vi "FPGA IO.vi"() -> ()   [LabVIEW 2013]
uses:
  Reusable/PAS/Main/Controls/Laser Modulation.ctl
  <vilib>/rvi/eio/common/nirviEmuClasses.ctl
  <vilib>/Platform/TimedLoop/XDataNode/timing_clust.ctl
  <vilib>/Platform/TimedLoop/XDataNode/nitl_modes.ctl
  <vilib>/Platform/TimedLoop/XDataNode/wakeup.ctl
  <vilib>/rvi/FXPMathLib/basic elements/FxpIntAccumulator/subVIs/nifxpmath_IntAccumulator_SimConfig.ctl
  <vilib>/rvi/Emulation/niFpgaSctlEmulationGetInTimedLoop.vi
  <vilib>/rvi/Emulation/niFpgaEmulationReportErrorSimple.vi
  <vilib>/rvi/Emulation/niFpgaGetClockAttributes.vi
  <vilib>/rvi/eio/common/nirviEmuTemplateMethod_errors.vi
  <vilib>/rvi/Emulation/niFpgaProcessEmulError.vi
  <vilib>/rvi/DataTransferAndStorage/Register/Emulation/niFpgaRegisterEmulationFpgaImpl.vi
  <instcachedir>/0/niFpgaRegisterEmulationFpgaImpl_DCF4BC0110594B98B44A971D60CEEC4D.lvgen/niFpgaRegisterEmulationFpgaImpl_DCF4BC0110594B98B44A971D60CEEC4D_001.vi
  <vilib>/rvi/DataTransferAndStorage/Container/Common/niFpgaContainerGetUniqueNameForEmu.vi
  <vilib>/rvi/Emulation/niFpgaCriticalErrorInLSC.vi
  <vilib>/rvi/FXPMathLib/basic elements/FxpIntAccumulator/simVIs/DllFxpIntAccumulator_sub.vi
  <vilib>/eio/EIOGrowableMethodNode/genericMethod/EIOGrowableMethodNode.xnode
  <vilib>/rvi/eio/nirviEIOMethodImplementation/nirviEIOMethodImplementation.xnode
  <vilib>/rvi/eio/nirviErrorMerge/nirviErrorMerge.xnode
  <vilib>/rvi/DataTransferAndStorage/Container/XNode/niFpgaContainer.xnode
  <vilib>/rvi/DataTransferAndStorage/Register/Emulation/niFpgaRegisterEmulation.vi
  <vilib>/rvi/FXPMathLib/FxpMul/XNode/nifxpmath_Multiplier.xnode
  <vilib>/rvi/FXPMathLib/FxpAdd/XNode/nifxpmath_Add.xnode
  <vilib>/eio/EIONode/EIONode.xnode
  <vilib>/Platform/TimedLoop/XDataNode/XDataNode.xnode
  <vilib>/rvi/FXPMathLib/basic elements/FxpIntAccumulator/XNode/nifxpmath_IntAccumulator.xnode
  <vilib>/rvi/FXPMathLib/basic elements/FxpDiscreteDelay/XNode/nifxpmath_DiscreteDelay.xnode
  <vilib>/rvi/FXPMathLib/sim/FxpSim.dll
  <vilib>/Platform/TimedLoop/XDataNode/XDNodeRunTimeDep.lvlib
panel:
  out "PAS AO":i16
  in  "Wave":T2={"f0"=3.2499898225069046e-05, "Mod"=enum."Sine", "hrange"=0.9999999997671694, "Offset"=0} {"f0" format="%.3g"}
  in  "Speaker":cluster{"Voltage":fxp<+,14,1>, "Offset":i16}={"Voltage"=1.0, "Offset"=0}
  out "HK Data":fxp<+/-,16,5>[](array[numeric])
  out "Valves In":u8
  in  "Enables":u8
  in  "Valves Out":u8
  in  "Stop":bool
  out "Timed Out":bool
  out "Stopped":bool
  out "Error Out":errorcluster
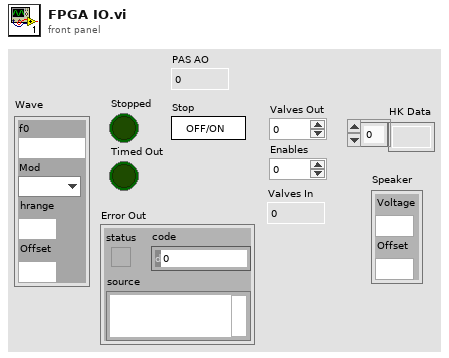
[diagram p1: front panel]
types:
  T1 = typedef "Laser Modulation.ctl" = enum8{"Sine", "Square"}
  T2 = cluster{"f0":fxp<+,32,0>, "Mod":T1, "hrange":fxp<+,32,0>, "Offset":i16}
  T3 = typedef "nirviEmuClasses.ctl" = enum16{"IO Read", "IO Write", "Method", "Property Read", "Property Write"}
  T4 = typedef "XDNodeRunTimeDep.lvlib/timing_clust.ctl" = cluster{"Expected End [f-1]":u64, "Actual End [f-1]":u64, "Finished Late? [f-1]":bool, "Expected End [i-1]":u64, "Actual End [i-1]":u64, "Finished Late? [i-1]":bool, "Expected Start [i]":u64, "Actual Start [i]":u64, "Expected Start [f]":u64, "Actual Start [f]":u64, "Source Name":string, "Structure Name":string, "Period":i64, "Deadline":i64, "Offset":i64, "Start":i64, "Priority":i32, "Timeout":i32, "Mode":T5, "Wakeup Reason":T6, "Error":errorcluster, "Source Type":string, "Secondary Source Type":string, "Global End Time":u64, "Global Start Time":u64, "Frame Duration":u64, "Iteration Duration":u64, "Assigned CPU":i32, "I/O Scan Engine Mode":u32}
  T5 = typedef "XDNodeRunTimeDep.lvlib/nitl_modes.ctl" = enum32{"No Change", "Process missed periods, maintain original phase", "Discard missed periods, maintain original phase", "Process missed periods, ignore original phase", "Discard missed periods, ignore original phase"}
  T6 = typedef "XDNodeRunTimeDep.lvlib/wakeup.ctl" = enum32{"Normal", "Aborted", "Asynchronous wakeup", "Timing source error", "Timed loop error", "Timeout"}
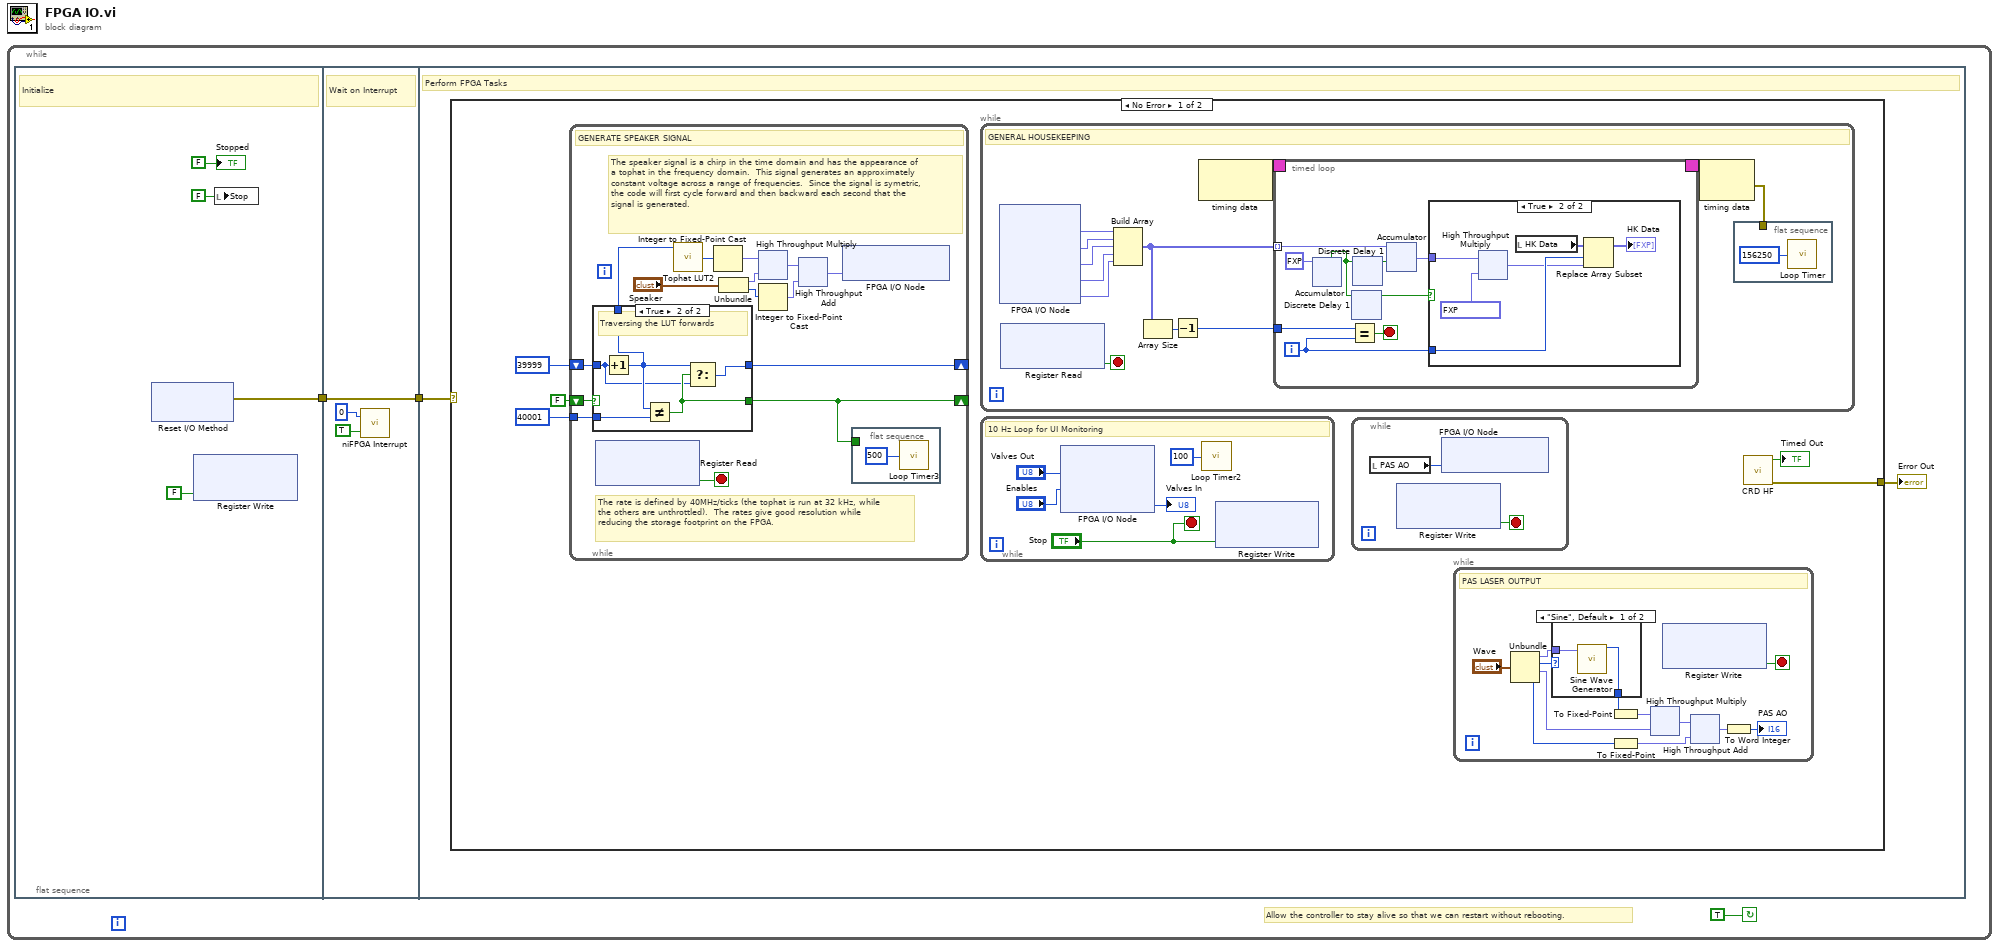
[diagram p0: block diagram]
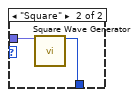
[diagram p2: hidden frame]
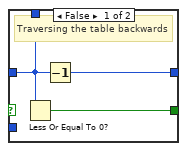
[diagram p3: hidden frame]
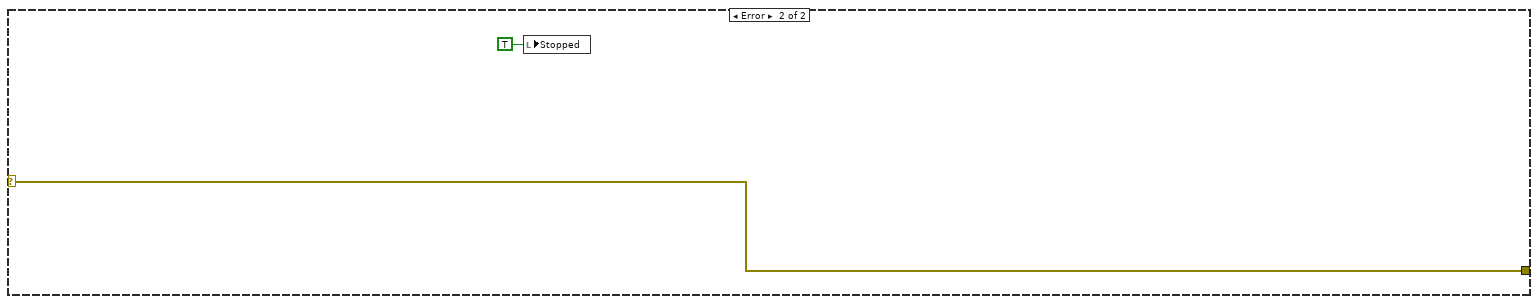
[diagram p5: hidden frame]
diagram:
  n1 = while {
    stop <- TRUE continue-if-true
    # "Allow the controller to stay alive so that we can restart without rebooting."
    n2 = flat-sequence {
      tunnel: [w6] -> w3
      tunnel: w3 -> [w52]
      tunnel: [w52] -> w2
      tunnel: w2 -> [w56]
      frame #0 {
        # "Initialize"
        n3 = xnode "Reset I/O Method"() -> ("error out"=w6:errorcluster)  [unwired: 2 in, 1 out]
        n4 = xnode ("Register Write")("Data"=FALSE) -> ()  [unwired: 1 in, 1 out]
        n5 = local write "Stop"(FALSE ("Stop")) -> ()
        "Stopped" <- FALSE ("Stopped")
      }
      frame #1 {
        # "Wait on Interrupt"
        n6 = call <vilib>:"niFPGA Interrupt.vi"("Wait Until Cleared (F)"=TRUE ("Wait Until Cleared"), "IRQ Number (0)"=u8 0 ("IRQ Number")) -> ()  [unwired: 1 in]
      }
      frame #2 {
        # "Perform FPGA Tasks"
        n7 = case shown="No Error" w56 {
          selector: w56 -> [_ w196]
          tunnel: [w61 w196] -> w55
          frame No Error {
            n8 = while {
              shift-right: [w82] -> _
              shift-left: FALSE -> [w94]
              shift-right: [w83] -> _
              shift-left: u16 39999 -> [w84]
              tunnel: u16 40001 ("y") -> [w85]
              stop <- w81 stop-if-true
              # "The rate is defined by 40MHz/ticks (the tophat is run at 32 kHz, while the others are unthrottled).  The rates give good resolution while reducing the storage footprint on the FPGA."
              # "The speaker signal is a chirp in the time domain and has the appearance of a tophat in the frequency domain.  This signal generates an approximately constant voltage across a range of frequencies.  Since the signal is symetric, the code will first cycle forward and then backward each second that the signal is generated."
              # "GENERATE SPEAKER SIGNAL"
              n9 = case "Check where we are in the chirp" shown="True" w94 {
                tunnel: w84 -> [w98 w99]
                tunnel: [w97 w102] -> w82
                tunnel: [w96 w103] -> w89
                tunnel: w85 -> [_ w101]
                tunnel: [w96 w100] -> w83
                frame False {
                  # "Traversing the table backwards"
                  n10 = Decrement(x=w98) -> (x-1=w96:u16)
                  n11 = Less Or Equal To 0?(x=w96) -> (x <= 0?=w97:bool)
                }
                frame True {
                  # "Traversing the LUT forwards"
                  n12 = Increment(x=w99) -> (x+1=w103:u16)
                  n13 = Not Equal?(x=w103, y=w101) -> (x != y?=w102:bool)
                  n14 = Select(t=w103, s=w102, f=w99) -> (s? t:f=w100:u16)
                }
              }
              n15 = xnode ("Register Read")() -> ("Data"=w81:bool)  [unwired: 1 in, 1 out]
              n16 = call "Tophat LUT2"("address"=w89) -> ("data out"=w91:i16)  [unwired: 8 in]
              n17 = Integer to Fixed-Point Cast(integer=w91) -> (fixed-point=w90:fxp<+/-,16,16>)  [unwired: 1 in]
              n18 = Unbundle("Speaker") -> ("Voltage"=w88:fxp<+,14,1>, "Offset"=w87:i16)
              n19 = xnode ("High Throughput Multiply")("x"=w90, "y"=w88) -> ("x*y"=w93:fxp<+/-,30,17>)
              n20 = Integer to Fixed-Point Cast(integer=w87) -> (fixed-point=w92:fxp<+/-,16,16>)  [unwired: 1 in]
              n21 = xnode ("High Throughput Add")("x"=w93, "y"=w92) -> ("x+y"=w80:fxp<+/-,20,5>)
              n22 = xnode "FPGA I/O Node"("PAS AO/AO1"=w80) -> ()  [unwired: 1 in, 1 out]
              n23 = flat-sequence {
                tunnel: w82 -> [_]
                frame #0 {
                  n24 = call "Loop Timer3"("Count(Ticks)"=u32 500) -> ()  [unwired: 1 out]
                }
              }
            }
            n25 = while {
              stop <- w108 stop-if-true
              # "GENERAL HOUSEKEEPING"
              n26 = xnode "FPGA I/O Node"() -> ("Tcomp"=w109:fxp<+/-,26,5>, "TEC hot"=w110:fxp<+/-,26,5>, "Troom"=w111:fxp<+/-,26,5>, "Box"=w112:fxp<+/-,26,5>, "Cell"=w113:fxp<+/-,26,5>)  [unwired: 5 in, 5 out]
              n27 = xnode ("Register Read")() -> ("Data"=w108:bool)  [unwired: 1 in, 1 out]
              n28 = Build Array(w109, w110, w111, w112, w113) -> (w107:fxp<+/-,26,5>[])
              n29 = Array Size(array=w107) -> (size(s)=w106:i32)
              n30 = Decrement(x=w106) -> (x-1=w105:i32)
              n31 = node-c288() -> (w115:T4)  [unwired: 1 in]
              n32 = timed-loop {
                timing: w115 -> [_]
                timing-out: [_] -> w114
                tunnel: w107 -> [w123] mode=indexing
                tunnel: w105 -> [w125]
                i -> [w117]
                stop <- w124 stop-if-true
                n33 = xnode "Accumulator"("x"=fxp<+,1,1> 1.0) -> ("carry-out/inverted borrow-out"=w120:bool)  [unwired: 4 in, 1 out]
                n34 = Equal?(x=w125, y=w117) -> (x = y?=w124:bool)
                n35 = xnode ("Discrete Delay 1")("D"=w120) -> ("Q"=w119:bool)
                n36 = xnode ("Discrete Delay 1")("D"=w120) -> ("Q"=w121:bool)
                n37 = xnode "Accumulator"("x"=w123, "load (F)"=w121) -> ("s"=w118:fxp<+/-,32,11>)  [unwired: 3 in, 1 out]
                n38 = case shown="True" w119 {
                  tunnel: w118 -> [_ w131]
                  tunnel: w117 -> [_ w129]
                  frame False {
                  }
                  frame True {
                    n39 = xnode ("High Throughput Multiply")("x"=w131, "y"=fxp<+,32,1> 0.00390625) -> ("x*y"=w128:fxp<+/-,16,5>)
                    n40 = local read "HK Data"() -> (w130:fxp<+/-,16,5>[])
                    n41 = Replace Array Subset(array=w130, new element=w128, index=w129) -> (→"HK Data":fxp<+/-,16,5>[])
                  }
                }
              }
              n42 = node-c288(w114) -> (w104:errorcluster)
              n43 = flat-sequence {
                tunnel: w104 -> [_]
                frame #0 {
                  n44 = call "Loop Timer"("Count(Ticks)"=u32 156250 ("Count(mSec)")) -> ()  [unwired: 1 out]
                }
              }
            }
            n45 = while {
              stop <- "Stop" stop-if-true
              # "10 Hz Loop for UI Monitoring"
              n46 = xnode "FPGA I/O Node"("Valves Out"="Valves Out", "Enables"="Enables") -> ("Valves In"=→"Valves In":u8)  [unwired: 3 in, 3 out]
              n47 = call "Loop Timer2"("Count(mSec)"=u32 100) -> ()  [unwired: 1 out]
              n48 = xnode ("Register Write")("Data"="Stop") -> ()  [unwired: 1 in, 1 out]
            }
            n49 = while {
              stop <- w79 stop-if-true
              n50 = local read "PAS AO"() -> (w78:i16)
              n51 = xnode ("Register Write")() -> ("Data"=w79:bool)  [unwired: 1 in, 1 out]
              n52 = xnode "FPGA I/O Node"("PAS AO/AO0"=w78) -> ()  [unwired: 1 in, 1 out]
            }
            n53 = while "Square wave generation - SCTL" {
              stop <- w73 stop-if-true
              # "PAS LASER OUTPUT"
              n54 = Unbundle("Wave") -> ("f0"=w71:fxp<+,32,0>, "Mod"=w70:T1, "hrange"=w67:fxp<+,32,0>, "Offset"=w65:i16)
              n55 = case shown="\"Sine\", Default" w70 {
                tunnel: w71 -> [w74 w77]
                tunnel: [w75 w76] -> w69
                frame "Sine", Default {
                  n56 = call "Sine Wave Generator"("frequency (periods/tick)"=w74) -> ("sine out"=w75:i16)  [unwired: 14 in]
                }
                frame "Square" {
                  n57 = call "Square Wave Generator"("frequency (periods/tick)"=w77) -> ("square wave out"=w76:i16)  [unwired: 14 in]
                }
              }
              n58 = To Fixed-Point(number=w69) -> (fixed-point=w68:fxp<+/-,16,16>)  [unwired: 1 in]
              n59 = To Fixed-Point(number=w65) -> (fixed-point=w64:fxp<+/-,16,16>)  [unwired: 1 in]
              n60 = xnode ("High Throughput Multiply")("x"=w68, "y"=w67) -> ("x*y"=w66:fxp<+/-,16,16>)
              n61 = xnode ("Register Write")() -> ("Data"=w73:bool)  [unwired: 1 in, 1 out]
              n62 = xnode ("High Throughput Add")("x"=w66, "y"=w64) -> ("x+y"=w63:fxp<+/-,16,16>)
              n63 = To Word Integer(number=w63) -> (16bit integer=→"PAS AO":i16)
            }
            n64 = call "CRD HF.vi"() -> ("error out"=w61:errorcluster, "Timed Out?"=→"Timed Out":bool)  [unwired: 10 in]
          }
          frame Error {
            n65 = local write "Stopped"(TRUE ("Stopped")) -> ()
          }
        }
        "Error Out" <- w55
      }
    }
  }
